vi "Stop.vi"(8 "error in (no error)":errorcluster, 11 "DelayLineLS4 in":refnum<class "DLLS4.lvclass">) -> (0 "error out":errorcluster, 3 "DelayLineLS4 out":refnum<class "DLLS4.lvclass">)   [LabVIEW 2015, in "DLLS4.lvclass"]
uses:
  DLLS4.lvclass
  GeneralFunctionality/GeneralFunctionality.lvclass/GeneralFunctionality.ctl
  GeneralFunctionality/GeneralFunctionality.lvclass
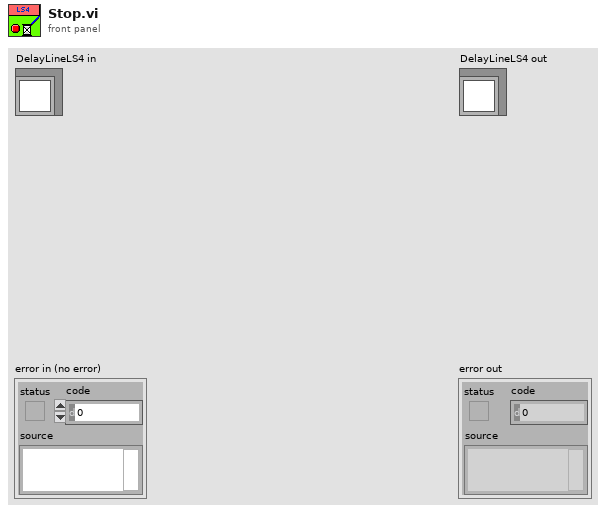
[diagram p1: front panel]
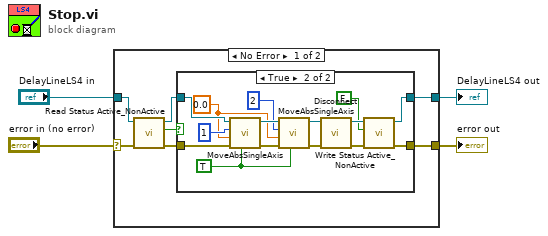
[diagram p0: block diagram]
diagram:
  n1 = case shown="No Error" "error in (no error)" {
    selector: "error in (no error)" -> [w7 w30]
    tunnel: [w11 w30] -> w2
    tunnel: [w10 w29] -> w3
    tunnel: "DelayLineLS4 in" -> [w9 w29]
    frame No Error {
      n2 = call "Read Status Active_NonActive.vi"("error in (no error)"=w7, "GeneralFunctionality in"=w9) -> ("error out"=w6:errorcluster, "Status Active/NonActive"=w5:bool, "GeneralFunctionality out"=w8:refnum<class "DLLS4.lvclass">)  [unwired: 7 in]
      n3 = case shown="True" w5 {
        tunnel: [w12 w27] -> w11
        tunnel: [w13 w28] -> w10
        tunnel: w8 -> [w13 w23]
        tunnel: w6 -> [w12 w18]
        frame False {
        }
        frame True {
          w14 = 0.0 ("Value")
          w17 = TRUE ("Wait")
          n4 = call-dynamic "MoveAbsSingleAxis.vi"("Wait"=w17, "error in (no error)"=w18, "Value"=w14, "Axis"=1, "DelayLineLS4 en entrée"=w23) -> ("error out"=w19:errorcluster, "DelayLineLS4 en sortie"=w22:refnum<class "DLLS4.lvclass">)  [unwired: 5 in]
          n5 = call-dynamic "MoveAbsSingleAxis.vi"("Wait"=w17, "error in (no error)"=w19, "Value"=w14, "Axis"=2, "DelayLineLS4 en entrée"=w22) -> ("error out"=w20:errorcluster, "DelayLineLS4 en sortie"=w21:refnum<class "DLLS4.lvclass">)  [unwired: 5 in]
          n6 = call "Disconnect.vi"("error in (no error)"=w20, "DelayLineLS4 en entrée"=w21) -> ("error out"=w26:errorcluster, "DelayLineLS4 out"=w25:refnum<class "DLLS4.lvclass">)  [unwired: 8 in]
          n7 = call "Write Status Active_NonActive.vi"("error in (no error)"=w26, "Status Active/NonActive"=FALSE, "GeneralFunctionality in"=w25) -> ("error out"=w27:errorcluster, "GeneralFunctionality out"=w28:refnum<class "DLLS4.lvclass">)  [unwired: 7 in]
        }
      }
    }
    frame Error {
    }
  }
  "error out" <- w2
  "DelayLineLS4 out" <- w3
